vi "_Client obtain occurance.vi"(8 "error in":errorcluster, 11 "Call ID in":T1) -> (0 "error out":errorcluster, 2 "occurrence":refnum<k4>, 3 "Call ID out":T1)   [LabVIEW 2021]
uses:
  <vilib>/gRPC/LabVIEW gRPC Library/Shared/grpcId.ctl
  <vilib>/Utility/error.llb/Error Cluster From Error Code.vi
  <vilib>/gRPC/LabVIEW gRPC Library/grpc-lvsupport-release.lvlib
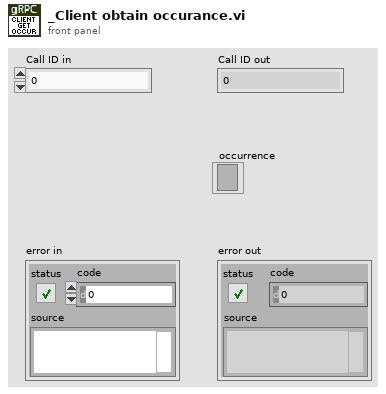
[diagram p1: front panel]
types:
  T1 = typedef "grpc-lvsupport-release.lvlib/grpcId.ctl" = u64
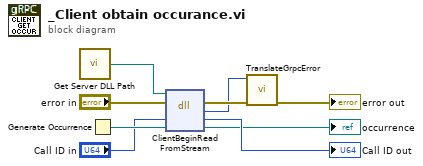
[diagram p0: block diagram]
diagram:
  n1 = call <vilib>:"Get Server DLL Path.vi"() -> ("Server dll path"=w3:path)
  n2 = Generate Occurrence() -> (w7:refnum<k4>)
  n3 = dll-call lib="?" fn="ClientBeginReadFromStream"(path in=w3, error in="error in", "ClientId"="Call ID in", "occurrence"=w7) -> (error out=w9:errorcluster, "return type"=w4:i32, "ClientId"=→"Call ID out":u64, "occurrence"=→"occurrence":refnum<k4>)  [unwired: 1 in, 1 out]
  n4 = call <vilib>:"TranslateGrpcError.vi"("error in"=w9, "Error Code"=w4) -> ("error out"=→"error out":errorcluster)  [unwired: 9 in]
